vi "mkGetSetFramerate.vi"(8 "Framerate":i32, 10 "Set? (F)":bool, 11 "IMAQ Refnum out":refnum<k11>) -> (0 "Framerate":i32, 1 "Maximum framerate":i32, 2 "Minimum framerate":i32, 3 "IMAQ Refnum (out)":refnum<k11>)   [LabVIEW 2011]
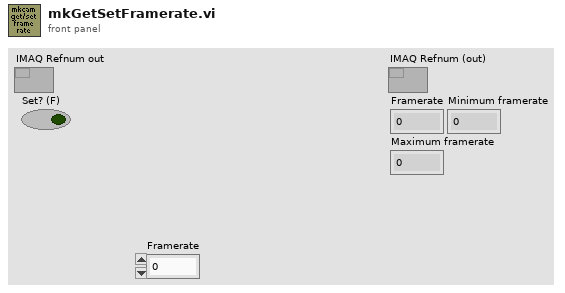
[diagram p1: front panel]
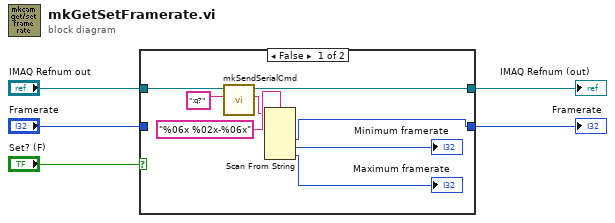
[diagram p0: block diagram]
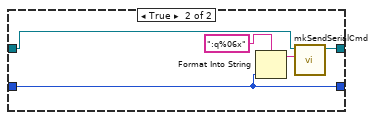
[diagram p2: hidden frame]
diagram:
  n1 = case shown="False" "Set? (F)" {
    tunnel: "IMAQ Refnum out" -> [w11 w18]
    tunnel: "Framerate" -> [_ w14]
    tunnel: [w6 w15] -> w2
    tunnel: [w9 w14] -> w1
    frame False {
      n2 = call "mkSendSerialCmd.vi"("String"=":q?", "IMAQ Refnum in"=w11) -> ("String Read"=w12:string, "IMAQ Refnum out"=w6:refnum<k11>)  [unwired: 6 in, 2 out]
      n3 = Scan From String(format string="%06x %02x-%06x", input string=w12) -> (output 1=w9:i32, output 2=→"Minimum framerate":i32, output 3=→"Maximum framerate":i32)  [unwired: 5 in, 3 out]
    }
    frame True {
      n4 = Format Into String(format string=":q%06x", w14) -> (resulting string=w16:string)  [unwired: 2 in, 1 out]
      n5 = call "mkSendSerialCmd.vi"("String"=w16, "IMAQ Refnum in"=w18) -> ("IMAQ Refnum out"=w15:refnum<k11>)  [unwired: 6 in, 3 out]
    }
  }
  "IMAQ Refnum (out)" <- w2
  "Framerate" <- w1
